vi "display_1s_stim_9s_ISI_CS1_CS2_CSmin_no_trigger.vi"() -> ()   [LabVIEW 2019]
uses:
  <vilib>/Analysis/Matrix/Datatypes/RealMatrix.ctl
  <vilib>/Utility/file.llb/Write Delimited Spreadsheet (DBL).vi
  <vilib>/Analysis/Matrix/NI_Matrix.lvlib
panel:
  out "ISI Time":dbl
  out "Stim TS":dbl
  out "Output":dbl[][](array[numeric])
  out "Output frame":T1
  out "Array temp1":T1
  out "Elapsed Time":dbl
  out "Display":bool=TRUE
  out "Trial":u32=1
  out "reward":dbl[](array[numeric])
  out "stim_id":dbl[](array[numeric])
  out "stim_loaded":dbl
  out "Timings":dbl[](array[numeric])
  out "Stimuli Loaded?":bool
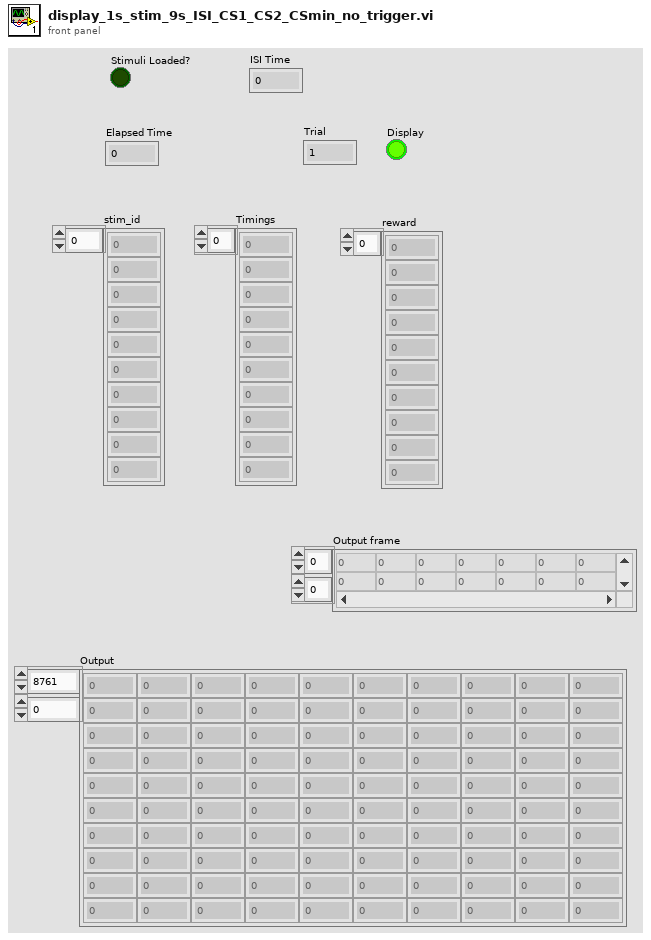
[diagram p1: front panel]
types:
  T1 = typedef "NI_Matrix.lvlib/RealMatrix.ctl" = dbl[][]
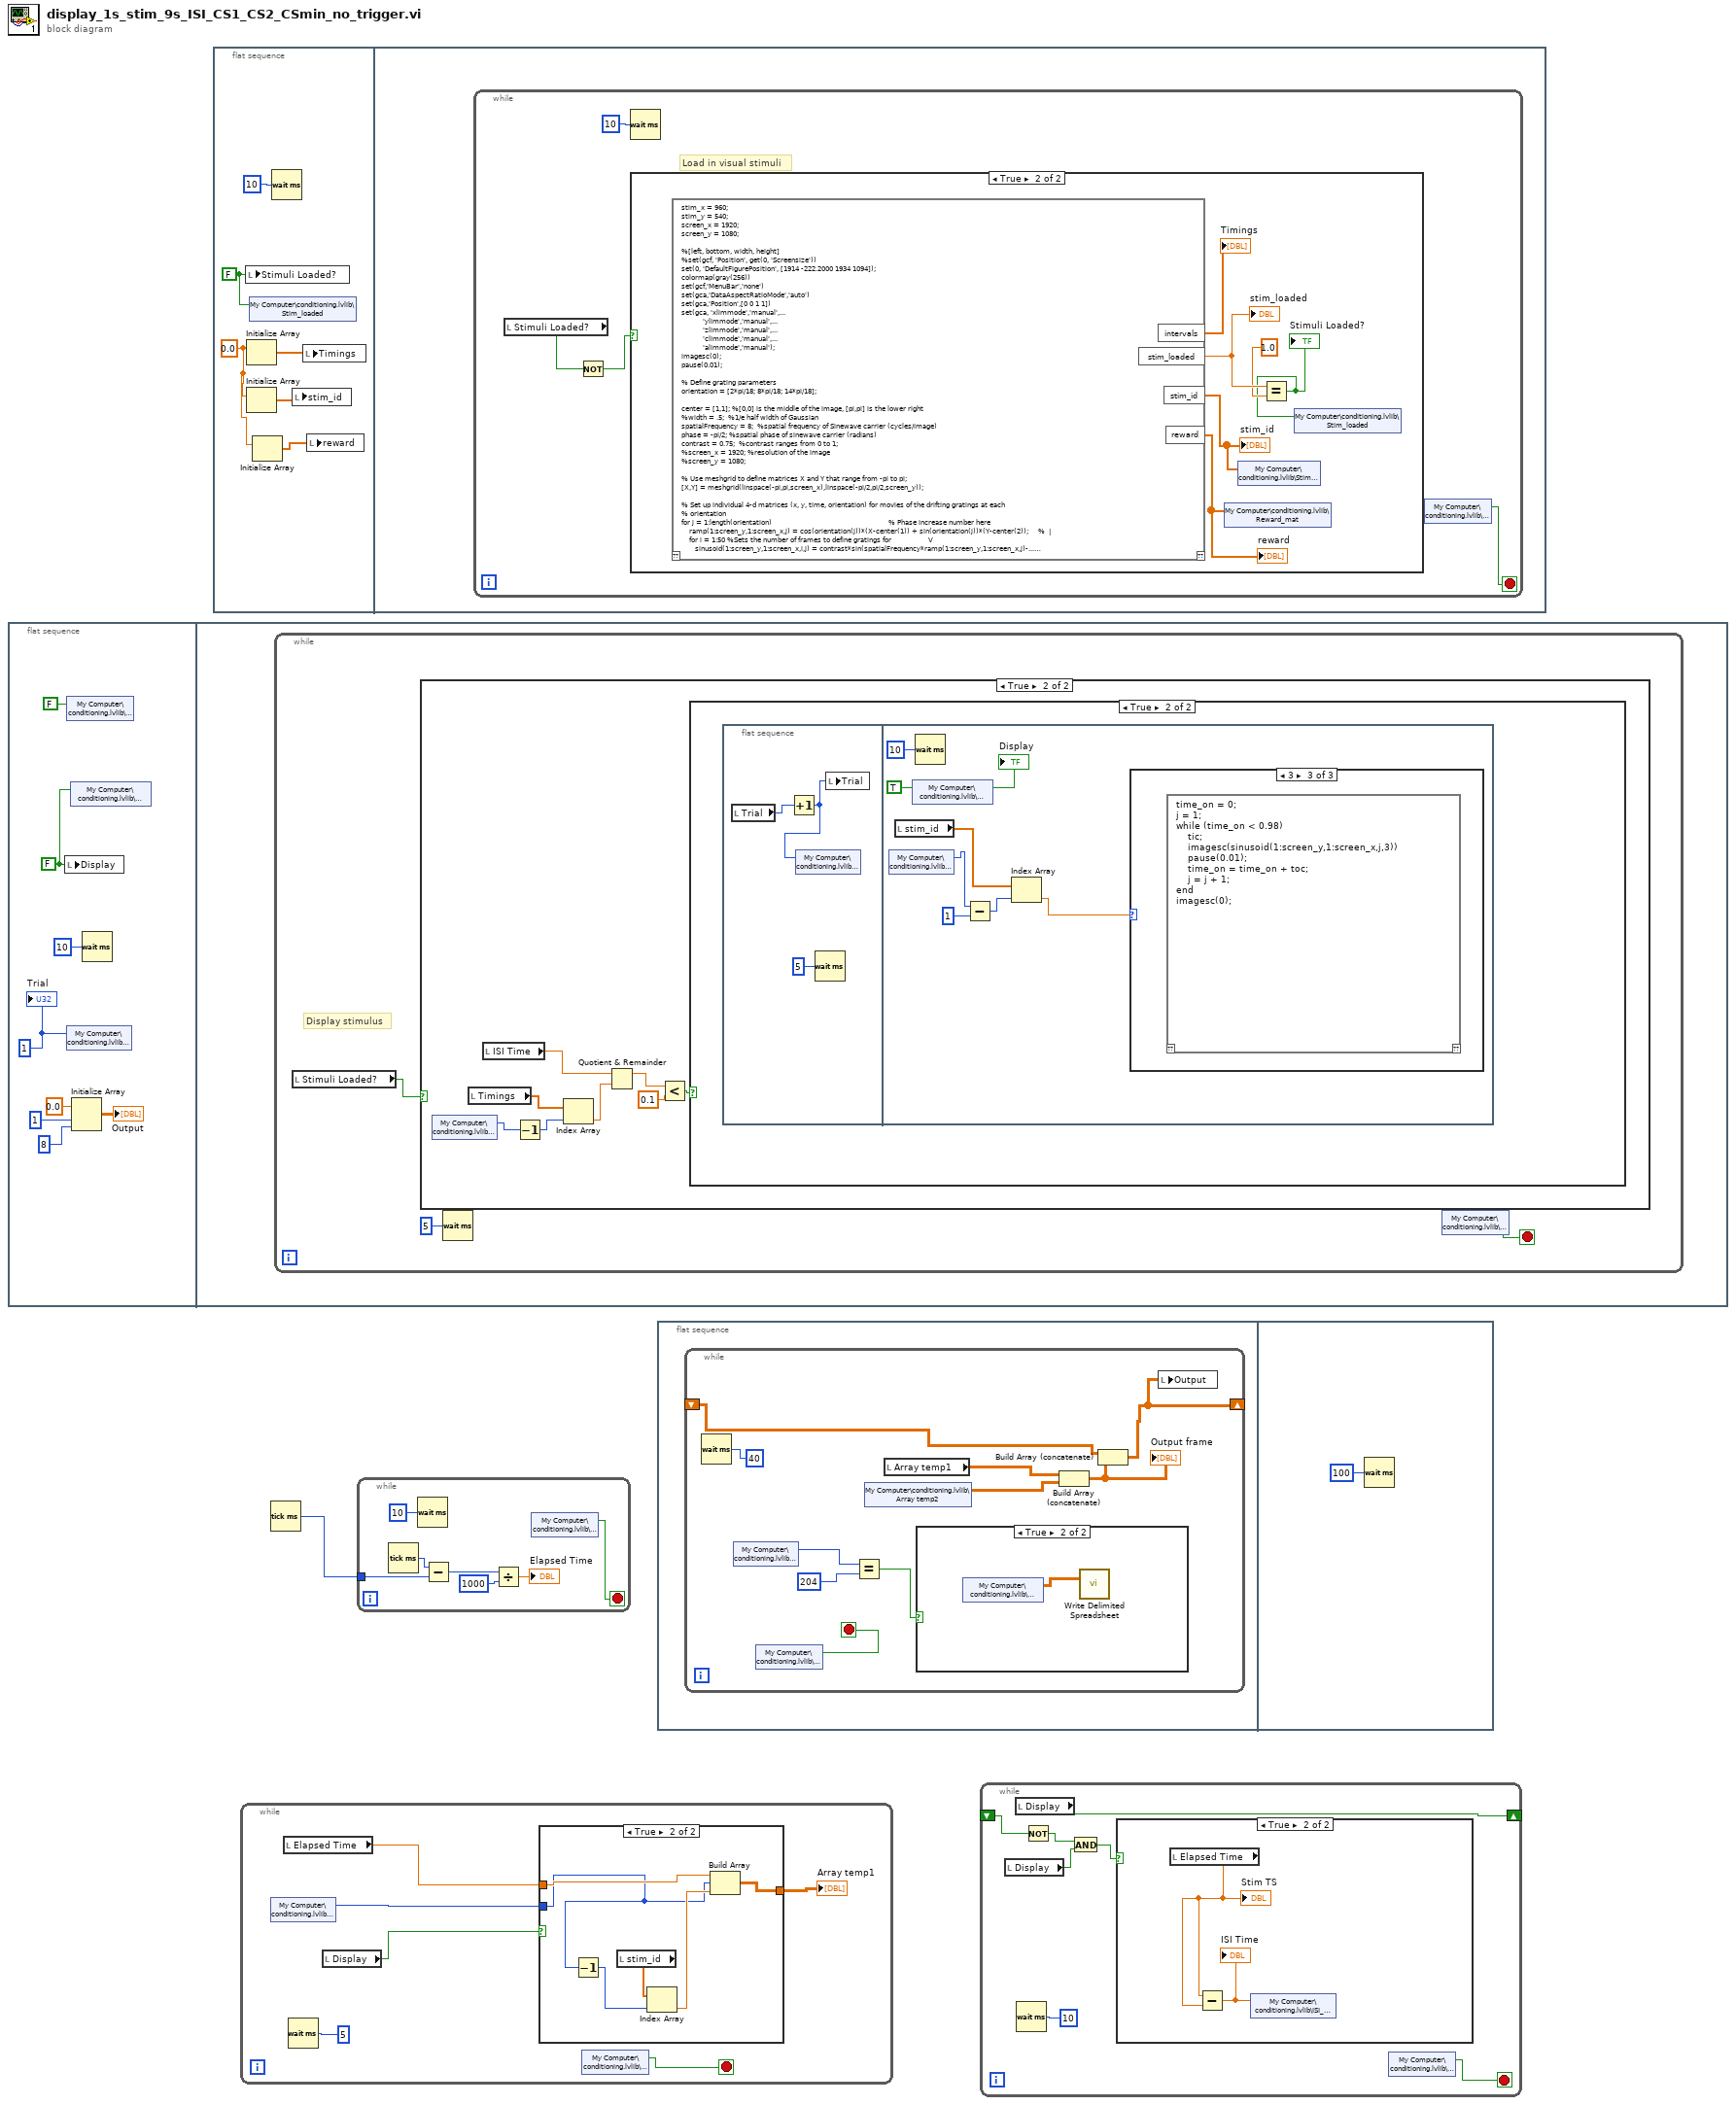
[diagram p0: block diagram]
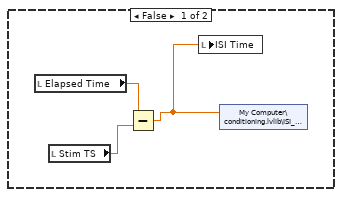
[diagram p2: hidden frame]
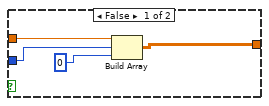
[diagram p3: hidden frame]
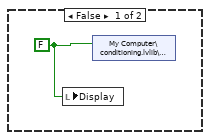
[diagram p7: hidden frame]
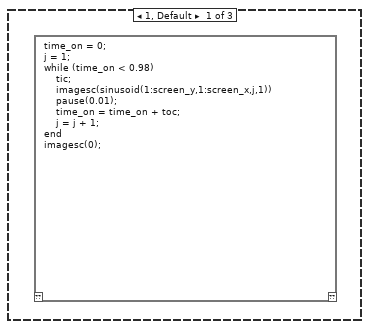
[diagram p8: hidden frame]
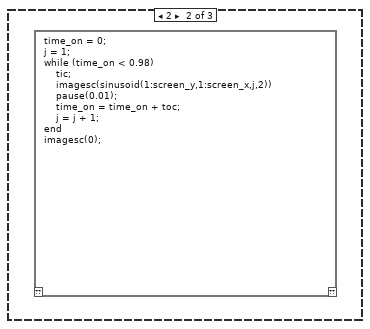
[diagram p9: hidden frame]
diagram:
  n1 = flat-sequence {
    frame #0 {
      w7 = FALSE ("Display")
      w9 = u32 1 ("Trial")
      n2 = local write "Display"(w7) -> ()
      n3 = shared-variable "My Computer\\conditioning.lvlib\\Stop"(FALSE ("Stop")) -> ()  [unwired: 1 in, 1 out]
      n4 = shared-variable "My Computer\\conditioning.lvlib\\Trial"(w9) -> ()  [unwired: 1 in, 1 out]
      n5 = shared-variable "My Computer\\conditioning.lvlib\\Display"(w7) -> ()  [unwired: 1 in, 1 out]
      n6 = Initialize Array(0.0 ("element"), 1 ("dimension size"), 8 ("dimension size")) -> (→"Output":dbl[][])
      n7 = Wait (ms)(milliseconds to wait=u32 10) -> ()  [unwired: 1 out]
      "Trial" <- w9
    }
    frame #1 {
      n8 = while {
        stop <- w11 stop-if-true
        # "Display stimulus"
        n9 = local read "Stimuli Loaded?"() -> (w10:bool)
        n10 = case shown="True" w10 {
          frame False {
          }
          frame True {
            n11 = shared-variable "My Computer\\conditioning.lvlib\\Trial"() -> (w16:u32)  [unwired: 1 in, 1 out]
            n12 = local read "Timings"() -> (w17:dbl[])
            n13 = local read "ISI Time"() -> (w13:dbl)
            n14 = Decrement(x=w16) -> (x-1=w15:u32)
            n15 = Index Array(array=w17, index=w15) -> (element=w14:dbl)
            n16 = Quotient & Remainder(x=w13, y=w14) -> (x-y*floor(x/y)=w20:dbl)  [unwired: 1 out]
            n17 = Less?(x=w20, y=0.1) -> (x < y?=w18:bool)
            n18 = case shown="True" w18 {
              frame False {
                w21 = FALSE ("Display")
                n19 = local write "Display"(w21) -> ()
                n20 = shared-variable "My Computer\\conditioning.lvlib\\Display"(w21) -> ()  [unwired: 1 in, 1 out]
              }
              frame True {
                n21 = flat-sequence {
                  frame #0 {
                    n22 = local read "Trial"() -> (w23:u32)
                    n23 = Increment(x=w23) -> (x+1=w22:u32)
                    n24 = shared-variable "My Computer\\conditioning.lvlib\\Trial"(w22) -> ()  [unwired: 1 in, 1 out]
                    n25 = Wait (ms)(milliseconds to wait=u32 5) -> ()  [unwired: 1 out]
                    n26 = local write "Trial"(w22) -> ()
                  }
                  frame #1 {
                    w29 = TRUE ("Boolean")
                    n27 = shared-variable "My Computer\\conditioning.lvlib\\Trial"() -> (w27:u32)  [unwired: 1 in, 1 out]
                    n28 = local read "stim_id"() -> (w30:dbl[])
                    n29 = shared-variable "My Computer\\conditioning.lvlib\\Display"(w29) -> ()  [unwired: 1 in, 1 out]
                    n30 = Wait (ms)(milliseconds to wait=u32 10) -> ()  [unwired: 1 out]
                    n31 = Subtract(x=w27, y=u32 1) -> (x-y=w28:u32)
                    n32 = Index Array(array=w30, index=w28) -> (element=w25:dbl)
                    n33 = case shown="3" w25 {
                      frame 1, Default {
                        n34 = script code="time_on = 0;\nj = 1;\nwhile (time_on < 0.98)\n    tic;\n    imagesc(sinusoid(1:screen_y,1:screen_x,j,1))\n    pause(0.01);\n    time_on = time_on + toc;\n    j = j + 1;\nend\nimagesc(0);"() -> ()  [unwired: 1 in, 1 out]
                      }
                      frame 2 {
                        n35 = script code="time_on = 0;\nj = 1;\nwhile (time_on < 0.98)\n    tic;\n    imagesc(sinusoid(1:screen_y,1:screen_x,j,2))\n    pause(0.01);\n    time_on = time_on + toc;\n    j = j + 1;\nend\nimagesc(0);"() -> ()  [unwired: 1 in, 1 out]
                      }
                      frame 3 {
                        n36 = script code="time_on = 0;\nj = 1;\nwhile (time_on < 0.98)\n    tic;\n    imagesc(sinusoid(1:screen_y,1:screen_x,j,3))\n    pause(0.01);\n    time_on = time_on + toc;\n    j = j + 1;\nend\nimagesc(0);"() -> ()  [unwired: 1 in, 1 out]
                      }
                    }
                    "Display" <- w29
                  }
                }
              }
            }
          }
        }
        n37 = Wait (ms)(milliseconds to wait=u32 5) -> ()  [unwired: 1 out]
        n38 = shared-variable "My Computer\\conditioning.lvlib\\Stop"() -> (w11:bool)  [unwired: 1 in, 1 out]
      }
    }
  }
  n39 = flat-sequence {
    frame #0 {
      w34 = 0.0 ("element")
      w32 = FALSE ("Stimuli Loaded?")
      n40 = local write "Stimuli Loaded?"(w32) -> ()
      n41 = Initialize Array(w34) -> (w36:dbl[])  [unwired: 1 in]
      n42 = Initialize Array(w34) -> (w35:dbl[])  [unwired: 1 in]
      n43 = shared-variable "My Computer\\conditioning.lvlib\\Stim_loaded"(w32) -> ()  [unwired: 1 in, 1 out]
      n44 = Initialize Array(w34) -> (w33:dbl[])  [unwired: 1 in]
      n45 = Wait (ms)(milliseconds to wait=u32 10) -> ()  [unwired: 1 out]
      n46 = local write "stim_id"(w35) -> ()
      n47 = local write "Timings"(w36) -> ()
      n48 = local write "reward"(w33) -> ()
    }
    frame #1 {
      n49 = while {
        stop <- w40 stop-if-true
        # "Load in visual stimuli"
        n50 = local read "Stimuli Loaded?"() -> (w39:bool)
        n51 = Not(x=w39) -> (.not. x?=w38:bool)
        n52 = Wait (ms)(milliseconds to wait=u32 10) -> ()  [unwired: 1 out]
        n53 = case shown="True" w38 {
          frame False {
          }
          frame True {
            n54 = script code="stim_x = 960;\nstim_y = 540;\nscreen_x = 1920;\nscreen_y = 1080;\n\n%[left, bottom, width, height]\n%set(gcf, 'Position', get(0, 'Screensize'))\nset(0, 'DefaultFigurePosition', [1914 -222.2000 1934 1094]);\ncolormap(gray(256))\nset(gcf,'MenuBar','none')\nset(gca,'DataAspectRatioMode','auto')\nset(gca,'Position',[0 0 1 1])\nset(gca, 'xlimmode','manual',...\n           'ylimmode','manual',...\n           'zlimmode','manual',...\n           'climmode','manual',...\n           'alimmode','manual');\nimagesc(0);\npause(0.01);\n\n% Define grating parameters\norientation = [2*pi/18; 8*pi/18; 14*pi/18];\n\ncenter = [1,1]; %[0,0] is the middle of the image, [pi,pi] is the lower right\n%width = .5;  %1/e half width of Gaussian\nspatialFrequency = 8;  %spatial frequency of Sinewave carrier (cycles/image)\nphase = -pi/2; %spatial phase of sinewave carrier (radians)\ncontrast = 0.75;  %contrast ranges from 0 to 1;\n%screen_x = 1920; %resolution of the image  \n%screen_y = 1080;\n\n% Use meshgrid to define matrices X and Y that range from -pi to pi;\n[X,Y] = meshgrid(linspace(-pi,pi,screen_x),linspace(-pi/2,pi/2,screen_y));\n\n% Set up individual 4-d matrices (x, y, time, orientation) for movies of the drifting gratings at each\n% orientation\nfor j = 1:length(orientation)                                                            % Phase increase number here\n    ramp(1:screen_y,1:screen_x,j) = cos(orientation(j))*(X-center(1)) + sin(orientation(j))*(Y-center(2));     %  |\n    for i = 1:50 %Sets the number of frames to define gratings for                   V\n       sinusoid(1:screen_y,1:screen_x,i,j) = contrast*sin(spatialFrequency*ramp(1:screen_y,1:screen_x,j)-...\n           (phase+(2*pi*(i-1)*(-30)/360))); %Number before '/360' sets the phase increase\n    end\nend\n\nintervals = [ones(1,41)*10 ones(1,41)*11 ones(1,41)*12 ones(1,41)*13 ones(1,40)*14];\nintervals = intervals(randperm(204));\nrand_idx = randperm(204);\nstim_id = [ones(1,34)*3 ones(1,34)*1 ones(1,34)*2 ones(1,34)*3 ones(1,34)*1 ones(1,34)*2];\nstim_id = stim_id(rand_idx);\nreward = [ones(1,34)*0 ones(1,34)*1 ones(1,34)*1 ones(1,34)*0 ones(1,34)*1 ones(1,34)*1];\nreward = reward(rand_idx);\n\nstim_loaded = 1;" ("Script Node")() -> ("stim_loaded"=w47:dbl, "intervals"=→"Timings":dbl[], "stim_id"=w42:dbl[], "reward"=w44:dbl[])  [unwired: 1 in, 1 out]
            "stim_loaded" <- w47
            "stim_id" <- w42
            "reward" <- w44
            n55 = shared-variable "My Computer\\conditioning.lvlib\\Reward_mat"(w44) -> ()  [unwired: 1 in, 1 out]
            n56 = shared-variable "My Computer\\conditioning.lvlib\\Stim_ID"(w42) -> ()  [unwired: 1 in, 1 out]
            n57 = Equal?(x=w47, y=1.0) -> (x = y?=w43:bool)
            "Stimuli Loaded?" <- w43
            n58 = shared-variable "My Computer\\conditioning.lvlib\\Stim_loaded"(w43) -> ()  [unwired: 1 in, 1 out]
          }
        }
        n59 = shared-variable "My Computer\\conditioning.lvlib\\Stop"() -> (w40:bool)  [unwired: 1 in, 1 out]
      }
    }
  }
  n60 = while {
    stop <- w48 stop-if-true
    n61 = shared-variable "My Computer\\conditioning.lvlib\\Trial"() -> (w50:u32)  [unwired: 1 in, 1 out]
    n62 = local read "Elapsed Time"() -> (w52:dbl)
    n63 = Wait (ms)(milliseconds to wait=u32 5) -> ()  [unwired: 1 out]
    n64 = local read "Display"() -> (w49:bool)
    n65 = case shown="True" w49 {
      tunnel: w50 -> [w56 w59]
      tunnel: w52 -> [w57 w61]
      tunnel: [w55 w62] -> w51
      frame False {
        n66 = Build Array(w57, w56, u32 0 ("milliseconds to wait")) -> (w55:T1)
      }
      frame True {
        n67 = Decrement(x=w59) -> (x-1=w58:u32)
        n68 = local read "stim_id"() -> (w63:dbl[])
        n69 = Index Array(array=w63, index=w58) -> (element=w60:dbl)
        n70 = Build Array(w61, w59, w60) -> (w62:T1)
      }
    }
    "Array temp1" <- w51
    n71 = shared-variable "My Computer\\conditioning.lvlib\\Stop"() -> (w48:bool)  [unwired: 1 in, 1 out]
  }
  n72 = Tick Count (ms)() -> (millisecond timer value=w1:u32)
  n73 = while {
    tunnel: w1 -> [w67]
    stop <- w64 stop-if-true
    n74 = Tick Count (ms)() -> (millisecond timer value=w68:u32)
    n75 = Wait (ms)(milliseconds to wait=u32 10) -> ()  [unwired: 1 out]
    n76 = Subtract(x=w68, y=w67) -> (x-y=w65:u32)
    n77 = Divide(x=w65, y=u32 1000) -> (x/y=→"Elapsed Time":dbl)
    n78 = shared-variable "My Computer\\conditioning.lvlib\\Stop"() -> (w64:bool)  [unwired: 1 in, 1 out]
  }
  n79 = flat-sequence {
    frame #0 {
      n80 = while {
        shift-right: [w77] -> _
        shift-left: _ -> [w78]
        stop <- w80 stop-if-true
        n81 = Wait (ms)(milliseconds to wait=u32 40) -> ()  [unwired: 1 out]
        n82 = shared-variable "My Computer\\conditioning.lvlib\\Trial"() -> (w73:u32)  [unwired: 1 in, 1 out]
        n83 = shared-variable "My Computer\\conditioning.lvlib\\Stop"() -> (w80:bool)  [unwired: 1 in, 1 out]
        n84 = Equal?(x=w73, y=u32 204) -> (x = y?=w71:bool)
        n85 = shared-variable "My Computer\\conditioning.lvlib\\Array temp2"() -> (w75:dbl[][])  [unwired: 1 in, 1 out]
        n86 = local read "Array temp1"() -> (w76:T1)
        n87 = case shown="True" w71 {
          frame False {
          }
          frame True {
            n88 = shared-variable "My Computer\\conditioning.lvlib\\Output"() -> (w81:dbl[][])  [unwired: 1 in, 1 out]
            n89 = call-poly <vilib>:"Write Delimited Spreadsheet.vi"("2D data"=w81) -> ()  [unwired: 13 in, 2 out]
          }
        }
        n90 = Build Array (concatenate)(w76, w75) -> (w74:T1)
        "Output frame" <- w74
        n91 = Build Array (concatenate) ("Build Matrix")(w78, w74) -> (w77:T1)
        n92 = local write "Output"(w77) -> ()
      }
    }
    frame #1 {
      n93 = Wait (ms)(milliseconds to wait=u32 100) -> ()  [unwired: 1 out]
    }
  }
  n94 = while {
    shift-right: [w87] -> _
    shift-left: _ -> [w86]
    stop <- w89 stop-if-true
    n95 = local read "Display"() -> (w84:bool)
    n96 = local read "Display"() -> (w87:bool)
    n97 = Wait (ms)(milliseconds to wait=u32 10) -> ()  [unwired: 1 out]
    n98 = Not(x=w86) -> (.not. x?=w85:bool)
    n99 = And(x=w85, y=w84) -> (x .and. y?=w83:bool)
    n100 = case shown="True" w83 {
      frame False {
        n101 = local read "Elapsed Time"() -> (w90:dbl)
        n102 = local read "Stim TS"() -> (w92:dbl)
        n103 = Subtract(x=w90, y=w92) -> (x-y=w91:dbl)
        n104 = local write "ISI Time"(w91) -> ()
        n105 = shared-variable "My Computer\\conditioning.lvlib\\ISI_Time"(w91) -> ()  [unwired: 1 in, 1 out]
      }
      frame True {
        n106 = local read "Elapsed Time"() -> (w93:dbl)
        "Stim TS" <- w93
        n107 = Subtract(x=w93, y=w93) -> (x-y=w94:dbl)
        "ISI Time" <- w94
        n108 = shared-variable "My Computer\\conditioning.lvlib\\ISI_Time"(w94) -> ()  [unwired: 1 in, 1 out]
      }
    }
    n109 = shared-variable "My Computer\\conditioning.lvlib\\Stop"() -> (w89:bool)  [unwired: 1 in, 1 out]
  }
